vi "Write CSV File_LV2012_NI Verified.vi"() -> ()   [LabVIEW 2017]
doc: "This example shows how to use the Write to Spreadsheet VI to write data to a Comma Separated Value (CSV) spreadsheet file which can be read in Microsoft Excel."
uses:
  <vilib>/Utility/file.llb/Write To Spreadsheet File (string).vi
  <vilib>/Utility/file.llb/Write To Spreadsheet File (DBL).vi
panel:
  in  "Channel Names":string[](array[string])=["Channel 1", "Channel 2", "Channel 3", "Channel 4", "Channel 5"]
  in  "Header Info":string[][](array[string])=[["Test Name", "Operator", "UUT"], ["Voltage", "National Instruments", "AA123"]]
  in  "File Name":path=path "C:/Documents and Settings/husmith/Desktop/CSVdata.csv"
  in  "Values to Write":i32=20
  in  "stop":bool
  in  "# of Channels":i32=5
  # "Overview: This example shows how to use the Write to Spreadsheet VI to write data to a Comma Separated Value (CSV) spreadsheet file which can be read in Microsoft Excel. \nRequirements: LabVIEW 2012 (or compatible)\nInstructions:\n1.  Choose where you would like to store the file\n2. Write the file properties such as the file header and the channel names\n3. Configure the number of channels and the number of samples/channel you want to generate\n4. Run the VI"
  # "File Properties"
  # "Generate Data"
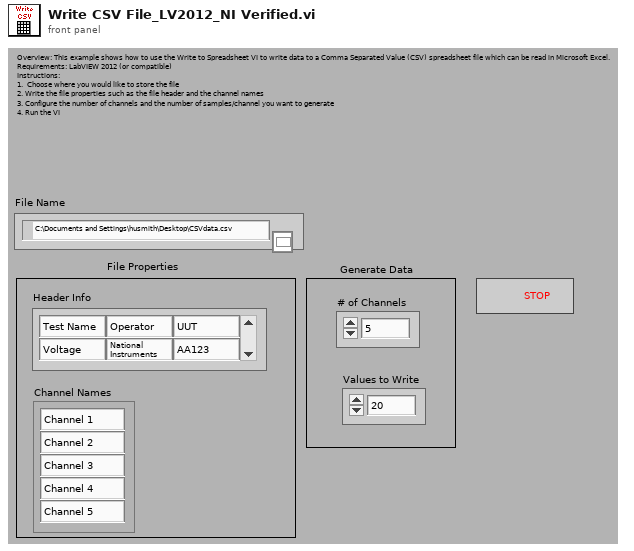
[diagram p1: front panel]
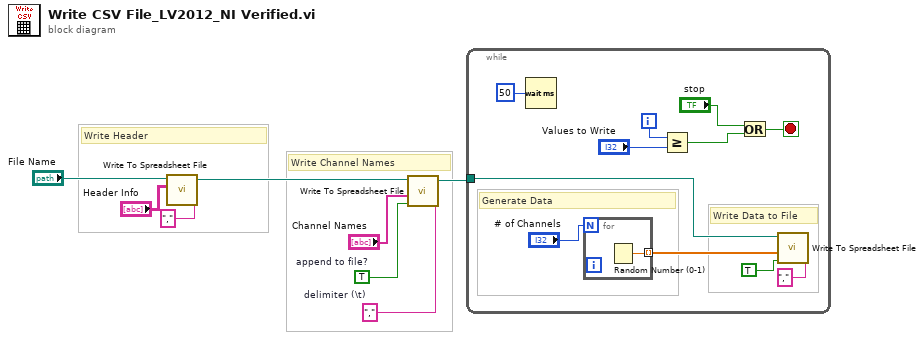
[diagram p0: block diagram]
diagram:
  w4 = TRUE  # append to file?
  w5 = ","  # delimiter (\t)
  # "Write Header"
  # "Write Channel Names"
  n1 = call-poly <vilib>:"Write To Spreadsheet File.vi"("delimiter (\\t)"="," ("delimiter (\\t)"), "2D data"="Header Info", "file path (dialog if empty)"="File Name") -> ("new file path (Not A Path if cancelled)"=w6:path)  [unwired: 4 in, 1 out]
  n2 = call-poly <vilib>:"Write To Spreadsheet File.vi"("delimiter (\\t)"=w5, "append to file? (new file:F)"=w4, "1D data"="Channel Names", "file path (dialog if empty)"=w6) -> ("new file path (Not A Path if cancelled)"=w8:path)  [unwired: 3 in, 1 out]
  n3 = while {
    tunnel: w8 -> [w11]
    i -> [w16]
    stop <- w13 stop-if-true
    # "Write Data to File"
    # "Generate Data"
    n4 = Wait (ms)(milliseconds to wait=u32 50 ("millisecond multiple")) -> ()  [unwired: 1 out]
    n5 = for {
      N: "# of Channels" -> [_]
      tunnel: [w20] -> w12 mode=indexing
      n6 = Random Number (0-1)() -> (number: 0 to 1=w20:dbl)
    }
    n7 = Greater Or Equal?(x=w16, y="Values to Write") -> (x >= y?=w14:bool)
    n8 = Or(x="stop", y=w14) -> (x .or. y?=w13:bool)
    n9 = call-poly <vilib>:"Write To Spreadsheet File.vi"("delimiter (\\t)"="," ("delimiter (\\t)"), "append to file? (new file:F)"=TRUE, "1D data"=w12, "file path (dialog if empty)"=w11) -> ()  [unwired: 3 in, 2 out]
  }
